vi "SetTaskChecked.vi"(8 "error in (no error)":errorcluster, 10 "TaskChecked":bool[](array[boolean]), 11 "TaskList in":refnum<class "TaskList.lvclass">) -> (0 "error out":errorcluster, 3 "TaskList out":refnum<class "TaskList.lvclass">)   [LabVIEW 2021, in "LvMarkdown.lvlib" / "TaskList.lvclass"]
uses:
  TaskList.lvclass
  TaskList.lvclass/TaskList.ctl
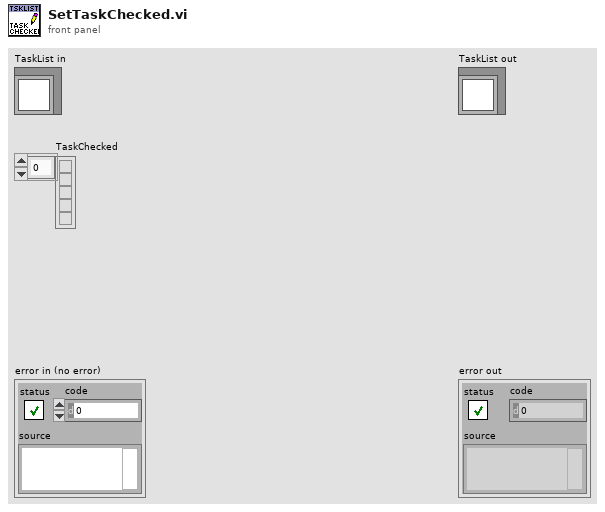
[diagram p1: front panel]
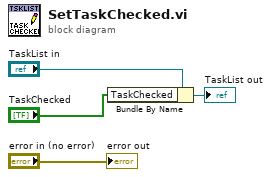
[diagram p0: block diagram]
diagram:
  n1 = Bundle By Name(cluster="TaskList in", "TaskChecked"="TaskChecked") -> (→"TaskList out":refnum<class "TaskList.lvclass">)
  "error out" <- "error in (no error)"
